vi "prep state ui.vi"(4 "Output Tag":refnum<vi>, 6 "Input Tag":refnum<vi>, 7 "Initial State":refnum<vi>, 8 "error in":errorcluster, 10 "engine configuration in":refnum<class "engine configuration.lvclass">, 11 "user tag bus module configuration in":refnum<class "fixed channel tag bus module configuration.lvclass">) -> (0 "error out":errorcluster, 2 "engine configuration out":refnum<class "engine configuration.lvclass">, 3 "user tag bus module configuration out":refnum<class "fixed channel tag bus module configuration.lvclass">)   [LabVIEW 2013, in "fixed channel tag bus module editor node.lvclass"]
uses:
  fixed channel tag bus module editor node.lvclass
  module/configuration/fixed channel tag bus module configuration.lvclass
  <vilib>/NI/Module Execution Interface/Engine Configuration/engine configuration.lvclass
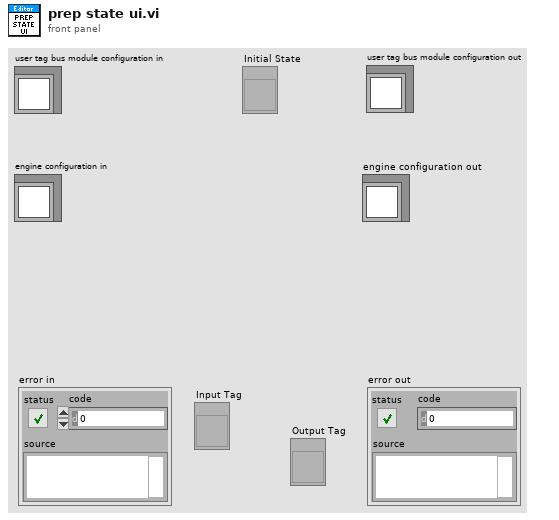
[diagram p1: front panel]
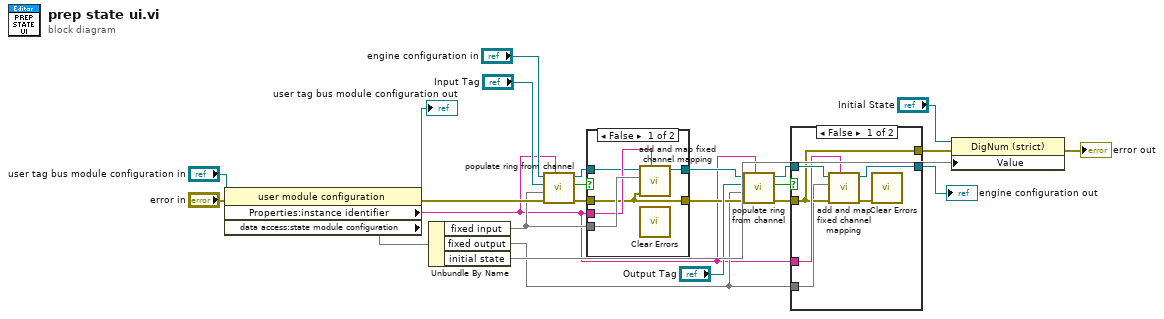
[diagram p0: block diagram]
diagram:
  n1 = property class="user module configuration"(reference="user tag bus module configuration in", error in="error in") -> (reference out=→"user tag bus module configuration out":refnum<class "fixed channel tag bus module configuration.lvclass">, error out=w20:errorcluster, "Properties:instance identifier"=w6:string, "data access:state module configuration"=w21)
  n2 = Unbundle By Name(w21) -> ("fixed input"=w10, "fixed output"=w7, "initial state"=w15)
  n3 = call "populate ring from channel.vi"("instance id"=w6, "error in"=w20, "channel"=w10, "ring"="Input Tag", "engine configuration in"="engine configuration in") -> ("error out"=w9:errorcluster, "mapped"=w13:bool, "engine configuration out"=w11:refnum<class "engine configuration.lvclass">)  [unwired: 4 in]
  n4 = case shown="False" w13 {
    tunnel: [w29 w31] -> w12
    tunnel: w11 -> [w26 w31]
    tunnel: w9 -> [w25 w30]
    tunnel: w10 -> [w28 _]
    tunnel: w6 -> [w27 _]
    tunnel: [w25 w30] -> w8
    frame False {
      n5 = call <vilib>:"add and map fixed channel mapping.vi"("module instance"=w27, "error in"=w25, "fixed channel"=w28, "engine configuration in"=w26) -> ("engine configuration out"=w29:refnum<class "engine configuration.lvclass">)  [unwired: 6 in, 1 out]
      n6 = call <vilib>:"Clear Errors.vi"() -> ()  [unwired: 7 in, 1 out]
    }
    frame True {
    }
  }
  n7 = call "populate ring from channel.vi"("instance id"=w6, "error in"=w8, "channel"=w7, "ring"="Output Tag", "engine configuration in"=w12) -> ("error out"=w3:errorcluster, "mapped"=w4:bool, "engine configuration out"=w5:refnum<class "engine configuration.lvclass">)  [unwired: 4 in]
  n8 = case shown="False" w4 {
    tunnel: [w32 w39] -> w2
    tunnel: w5 -> [w37 w39]
    tunnel: w3 -> [w35 w38]
    tunnel: w7 -> [w34 _]
    tunnel: w6 -> [w36 _]
    tunnel: [w35 w38] -> w1
    frame False {
      n9 = call <vilib>:"add and map fixed channel mapping.vi"("module instance"=w36, "error in"=w35, "fixed channel"=w34, "engine configuration in"=w37) -> ("error out"=w33:errorcluster, "engine configuration out"=w32:refnum<class "engine configuration.lvclass">)  [unwired: 6 in]
      n10 = call <vilib>:"Clear Errors.vi"("error in (no error)"=w33) -> ()  [unwired: 6 in, 1 out]
    }
    frame True {
    }
  }
  "engine configuration out" <- w2
  n11 = property class="DigNum (strict)"(reference="Initial State", error in=w1, "Value"=w15) -> (error out=→"error out":errorcluster)  [unwired: 1 out]
